vi "SaveSeqToXMLFile.vi"(8 "error in (no error)":errorcluster, 11 "Sequence in":refnum<class "Sequence.lvclass">) -> (0 "error out":errorcluster, 3 "Sequence out":refnum<class "Sequence.lvclass">)   [LabVIEW 2017]
uses:
  Sequence.lvclass
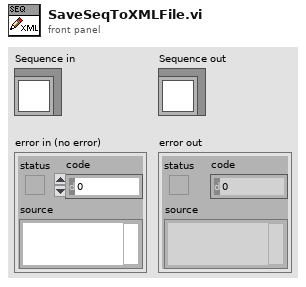
[diagram p1: front panel]
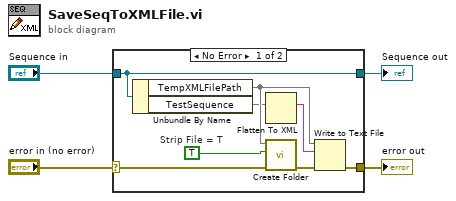
[diagram p0: block diagram]
diagram:
  n1 = case shown="No Error" "error in (no error)" {
    selector: "error in (no error)" -> [w8 w14]
    tunnel: [w10 w14] -> w3
    tunnel: [w12 w13] -> w1
    tunnel: "Sequence in" -> [w12 w13]
    frame No Error {
      w9 = TRUE  # Strip File = T
      n2 = Unbundle By Name(w12) -> ("TempXMLFilePath"=w6, "TestSequence"=w5)
      n3 = Flatten To XML(anything=w5) -> (xml string=w11:string)
      n4 = call "Create Folder.vi"("error in (no error)"=w8, "Strip File = T"=w9, "Path"=w6) -> ("error out"=w7:errorcluster)  [unwired: 8 in]
      n5 = Write to Text File(file (use dialog)=w6, text=w11, error in=w7) -> (error out=w10:errorcluster)  [unwired: 1 in, 2 out]
    }
    frame Error {
    }
  }
  "error out" <- w3
  "Sequence out" <- w1
